vi "Generate Data Frame Vectors.vi"(0 "RFFE RegReadExt Command in":refnum<class "RFFE RegReadExt Command.lvclass">, 11 "error in (no error)":errorcluster) -> (4 "RFFE RegReadExt Command out":refnum<class "RFFE RegReadExt Command.lvclass">, 6 "Data Frame Vectors":string[](array[string]), 15 "error out":errorcluster)   [LabVIEW 2018, in "MIPI RFFE API.lvlib" / "RFFE RegReadExt Command.lvclass"]
uses:
  RFFE RegReadExt Command.lvclass
  MIPI RFFE API.lvlib
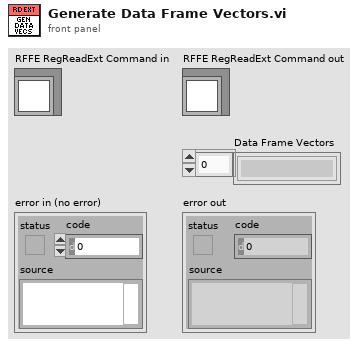
[diagram p1: front panel]
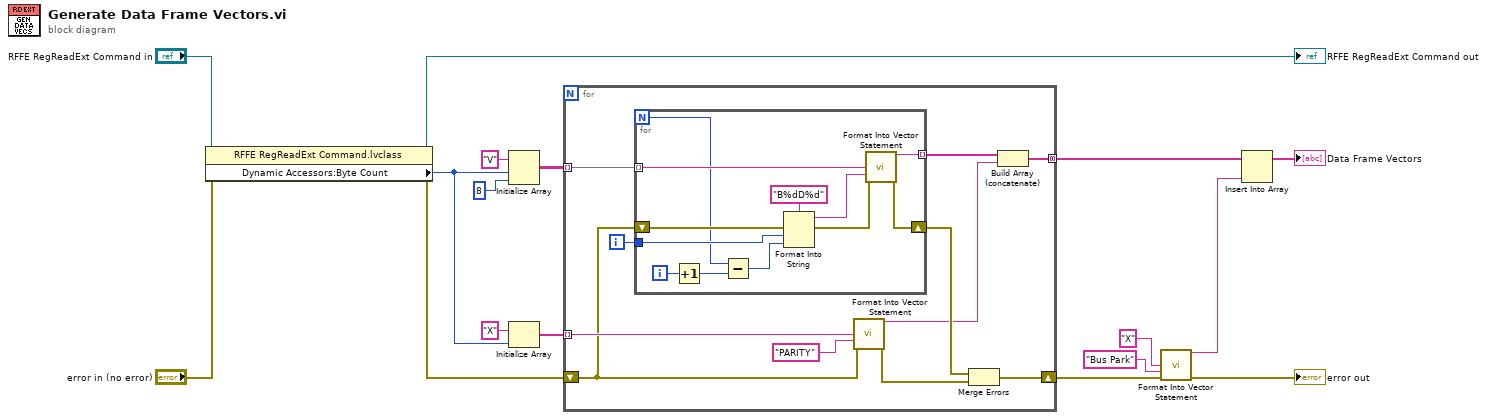
[diagram p0: block diagram]
diagram:
  n1 = property class="RFFE RegReadExt Command.lvclass"(reference="RFFE RegReadExt Command in", error in="error in (no error)") -> (reference out=→"RFFE RegReadExt Command out":refnum<class "RFFE RegReadExt Command.lvclass">, error out=w13:errorcluster, "Dynamic Accessors:Byte Count"=w11:i32)
  n2 = Initialize Array("V", w11, 8 ("y")) -> (w9:string[][])
  n3 = Initialize Array("X", w11) -> (w8:string[])
  n4 = for {
    shift-right: [w21] -> w6
    shift-left: w13 -> [w24]
    tunnel: w9 -> [w28] mode=indexing
    tunnel: w8 -> [w26] mode=indexing
    tunnel: [w18] -> w3 mode=concatenating
    i -> [w27]
    n5 = for {
      N -> [w31]
      tunnel: w28 -> [w40] mode=indexing
      shift-right: [w37] -> w23
      shift-left: w24 -> [w36]
      tunnel: w27 -> [w34]
      tunnel: [w33] -> w20 mode=indexing
      i -> [w32]
      n6 = Increment(x=w32) -> (x+1=w29:i32)
      n7 = Subtract(x=w31, y=w29) -> (x-y=w30:i32)
      n8 = Format Into String(format string="B%dD%d", error in=w36, w34, w30) -> (resulting string=w39:string, error out=w38:errorcluster)  [unwired: 1 in]
      n9 = call "Format Into Vector Statement.vi"("DATA (0)"=w40, "Comment"=w39, "error in (no error)"=w38) -> ("Vector Statement"=w33:string, "error out"=w37:errorcluster)  [unwired: 11 in]
    }
    n10 = call "Format Into Vector Statement.vi"("DATA (0)"=w26, "Comment"="PARITY", "error in (no error)"=w24) -> ("Vector Statement"=w19:string, "error out"=w22:errorcluster)  [unwired: 11 in]
    n11 = Merge Errors(w23, w22) -> (w21:errorcluster)
    n12 = Build Array (concatenate)(w20, w19) -> (w18:string[])
  }
  n13 = call "Format Into Vector Statement.vi"("DATA (0)"="X", "Comment"="Bus Park", "error in (no error)"=w6) -> ("Vector Statement"=w1:string, "error out"=→"error out":errorcluster)  [unwired: 11 in]
  n14 = Insert Into Array(array=w3, new element=w1) -> (→"Data Frame Vectors":string[])  [unwired: 1 in]
